vi "SSC Digital Burst Pattern.vi"(0 "Digital SSC in":T1[](array[typedef]), 1 "Start Label":string, 2 "select digital function?":bool=TRUE caption="select digital function? (T)", 3 "wait until done?":bool=TRUE caption="wait until done? (T)", 7 "timeout (s)":dbl=10.0, 11 "error in":errorcluster) -> (4 "Digital SSC out":T1[](array[typedef]), 15 "error out":errorcluster)   [LabVIEW 2020]
doc: "Uses the start label you specify to burst the pattern on the pin(s) and pin group(s) you specify."
uses:
  SSC Digital.ctl
  <instrlib>/niDigital/niDigital.llb/niDigital Burst Pattern (Burst Only).vi
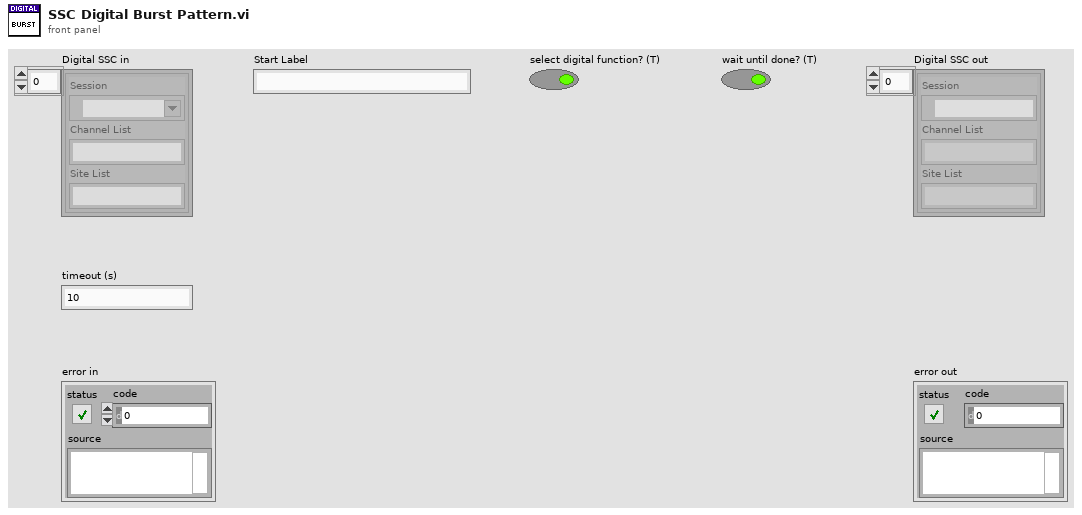
[diagram p1: front panel]
types:
  T1 = typedef "SSC Digital.ctl" = cluster{"Session":refnum<k15>, "Channel List":string, "Site List":string}
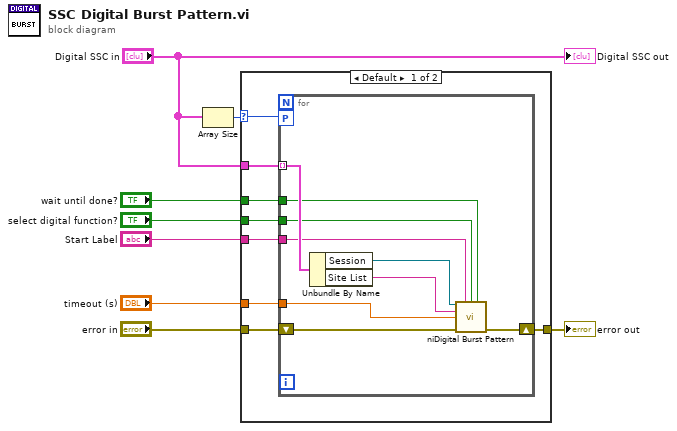
[diagram p0: block diagram]
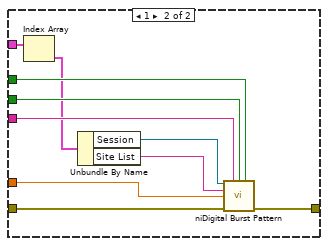
[diagram p2: hidden frame]
diagram:
  n1 = Array Size(array="Digital SSC in") -> (size(s)=w2:i32)
  n2 = case shown="Default" w2 {
    selector: w2 -> [w10 _]
    tunnel: "Start Label" -> [w16 w35]
    tunnel: "select digital function?" -> [w15 w34]
    tunnel: "wait until done?" -> [w14 w33]
    tunnel: "timeout (s)" -> [w13 w32]
    tunnel: "error in" -> [w12 w31]
    tunnel: [w11 w30] -> w3
    tunnel: "Digital SSC in" -> [w9 w29]
    frame Default {
      n3 = for {
        tunnel: w9 -> [w25] mode=indexing
        tunnel: w16 -> [w24]
        tunnel: w15 -> [w23]
        tunnel: w14 -> [w22]
        workers-P: w10 -> [_]
        tunnel: w13 -> [w19]
        shift-right: [w20] -> w11
        shift-left: w12 -> [w21]
        n4 = Unbundle By Name(w25) -> ("Session"=w18:refnum<k15>, "Site List"=w17:string)
        n5 = call-poly <instrlib>:"niDigital Burst Pattern.vi"("instrument handle"=w18, "start label"=w24, "select digital function? (T)"=w23, "wait until done? (T)"=w22, "site list"=w17, "timeout (s)"=w19, "error in"=w21) -> ("error out"=w20:errorcluster)  [unwired: 7 in, 1 out]
      }
    }
    frame 1 {
      n6 = Index Array(array=w29) -> (element=w26:T1)  [unwired: 1 in]
      n7 = Unbundle By Name(w26) -> ("Session"=w28:refnum<k15>, "Site List"=w27:string)
      n8 = call-poly <instrlib>:"niDigital Burst Pattern.vi"("instrument handle"=w28, "start label"=w35, "select digital function? (T)"=w34, "wait until done? (T)"=w33, "site list"=w27, "timeout (s)"=w32, "error in"=w31) -> ("error out"=w30:errorcluster)  [unwired: 7 in, 1 out]
    }
  }
  "error out" <- w3
  "Digital SSC out" <- "Digital SSC in"
